vi "getSample.vi"(10 "percentage":dbl, 11 "max":dbl) -> (3 "getSample":i32[](array[numeric]))   [LabVIEW 2014]
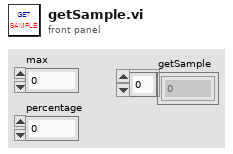
[diagram p1: front panel]
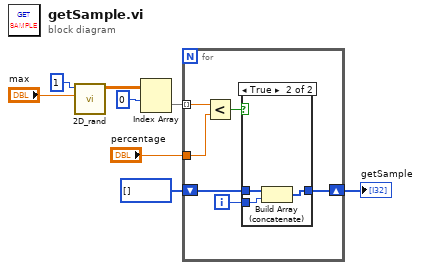
[diagram p0: block diagram]
diagram:
  n1 = call "2D_rand.vi"("column_number"="max", "row_number"=1) -> ("2D_Rand"=w6:dbl[][])  [unwired: 9 in]
  n2 = Index Array(array=w6, index (row)=0) -> (element=w4:dbl[])  [unwired: 1 in]
  n3 = for {
    tunnel: w4 -> [w14] mode=indexing
    tunnel: "percentage" -> [w13]
    shift-right: [w10] -> w1
    shift-left: i32[] [] -> [w9]
    i -> [w11]
    n4 = Less?(x=w14, y=w13) -> (x < y?=w12:bool)
    n5 = case shown="True" w12 {
      tunnel: w11 -> [_ w18]
      tunnel: [w15 w17] -> w10
      tunnel: w9 -> [w15 w16]
      frame False {
      }
      frame True {
        n6 = Build Array (concatenate)(w16, w18) -> (w17:i32[])
      }
    }
  }
  "getSample" <- w1
